vi "Action Runner.vi"(8 "error in (no error)":errorcluster, 9 "Message Data":variant, 10 "Message":string, 11 "Asynchronous Action In":refnum<class "Asynchronous Action.lvclass">) -> (0 "error out":errorcluster, 3 "Asynchronous Action Out":refnum<class "Asynchronous Action.lvclass">)   [LabVIEW 2020, in "Asynchronous Action.lvclass"]
uses:
  Asynchronous Action.lvclass
  Error Handler Interface/Error Handler Interface.lvclass
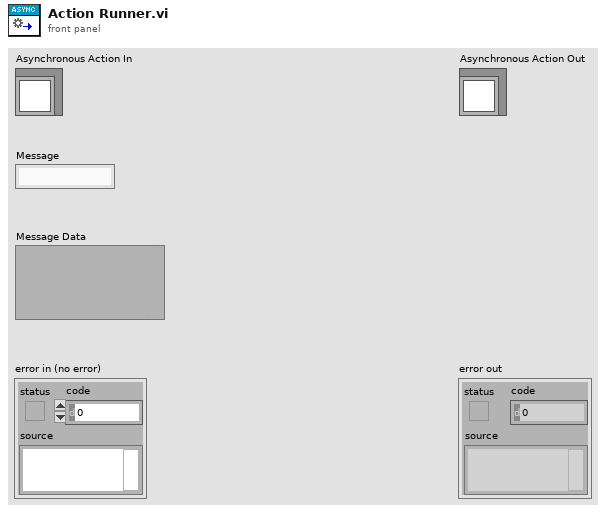
[diagram p1: front panel]
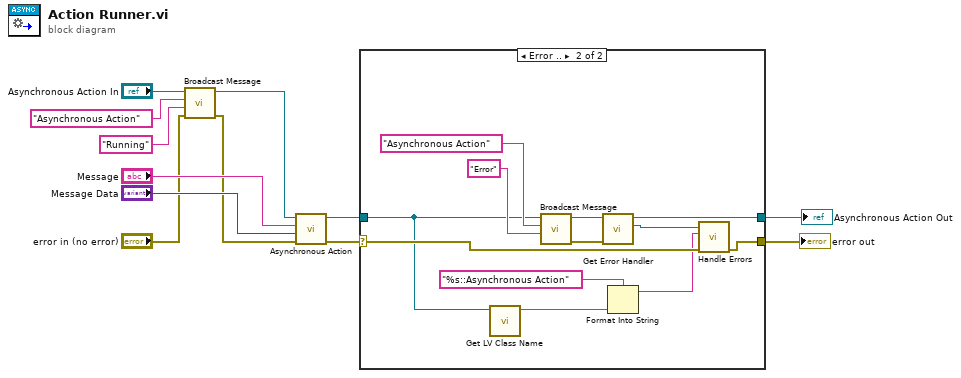
[diagram p0: block diagram]
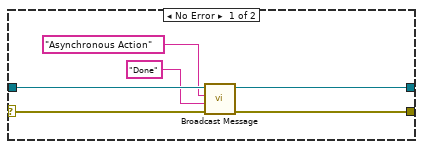
[diagram p2: hidden frame]
diagram:
  n1 = call-dynamic "Broadcast Message.vi"("error in (no error)"="error in (no error)", "Message Data"="Running" ("Message"), "Message"="Asynchronous Action", "Asynchronous Action In"="Asynchronous Action In") -> ("error out"=w3:errorcluster, "Asynchronous Action Out"=w6:refnum<class "Asynchronous Action.lvclass">)  [unwired: 6 in]
  n2 = call-dynamic "Asynchronous Action.vi"("error in (no error)"=w3, "Message Data"="Message Data", "Message"="Message", "Asynchronous Action In"=w6) -> ("error out"=w7:errorcluster, "Asynchronous Action Out"=w10:refnum<class "Asynchronous Action.lvclass">)  [unwired: 6 in]
  n3 = case shown="Error .." w7 {
    selector: w7 -> [w16 w30]
    tunnel: w10 -> [w17 w19]
    tunnel: [w18 w27] -> w9
    tunnel: [w15 w29] -> w8
    frame No Error {
      n4 = call-dynamic "Broadcast Message.vi"("error in (no error)"=w16, "Message Data"="Done" ("Message"), "Message"="Asynchronous Action", "Asynchronous Action In"=w17) -> ("error out"=w15:errorcluster, "Asynchronous Action Out"=w18:refnum<class "Asynchronous Action.lvclass">)  [unwired: 6 in]
    }
    frame Error {
      n5 = call <vilib>:"Get LV Class Name.vi"("object"=w19) -> ("class name"=w25:string)  [unwired: 9 in, 1 out]
      n6 = call-dynamic "Broadcast Message.vi"("Message Data"="Error" ("Message"), "Message"="Asynchronous Action", "Asynchronous Action In"=w19) -> ("error out"=w21:errorcluster, "Asynchronous Action Out"=w20:refnum<class "Asynchronous Action.lvclass">)  [unwired: 7 in]
      n7 = call-dynamic "Get Error Handler.vi"("error in (no error)"=w21, "Asynchronous Action In"=w20) -> ("Error Handler"=w28:refnum<class "Error Handler Interface.lvclass">, "Asynchronous Action Out"=w27:refnum<class "Asynchronous Action.lvclass">)  [unwired: 7 in, 1 out]
      n8 = Format Into String(format string="%s::Asynchronous Action", w25) -> (resulting string=w24:string)  [unwired: 2 in, 1 out]
      n9 = call-dynamic "Handle Errors.vi"("error in (no error)"=w30, "Location"=w24, "Error Handler Interface In"=w28) -> ("error out"=w29:errorcluster)  [unwired: 7 in, 1 out]
    }
  }
  "error out" <- w8
  "Asynchronous Action Out" <- w9
